vi "Actor Core.vi"(0 "MainUI in":refnum<class "MainUI.lvclass">, 11 "Error in":errorcluster caption="Error in (no error)") -> (4 "MainUI out":refnum<class "MainUI.lvclass">, 15 "Error out":errorcluster)   [LabVIEW 2018, in "HOG MainUI.lvlib" / "MainUI.lvclass"]
doc: "GPower Actor Core VI.\n\nSteen Schmidt\nGPower\n9/9 2018"
uses:
  MainUI.lvclass
  <vilib>/GPower/Actor/Library/Actor Class/Actor.lvclass
  <vilib>/GPower/Actor/Library/Responder Class/Responder.lvclass
  C:/Program Files (x86)/National Instruments/LabVIEW 2018/vi.lib/GPower/Actor/Library/Actor Class/Actor.lvclass
  <vilib>/GPower/UI/Library/GP UI.lvlib
  <vilib>/GPower/UI/Library/Controls/Clear Control/Clear Table.vi
panel:
  in  "MemberList":i32(listbox)
  in  "Search":string
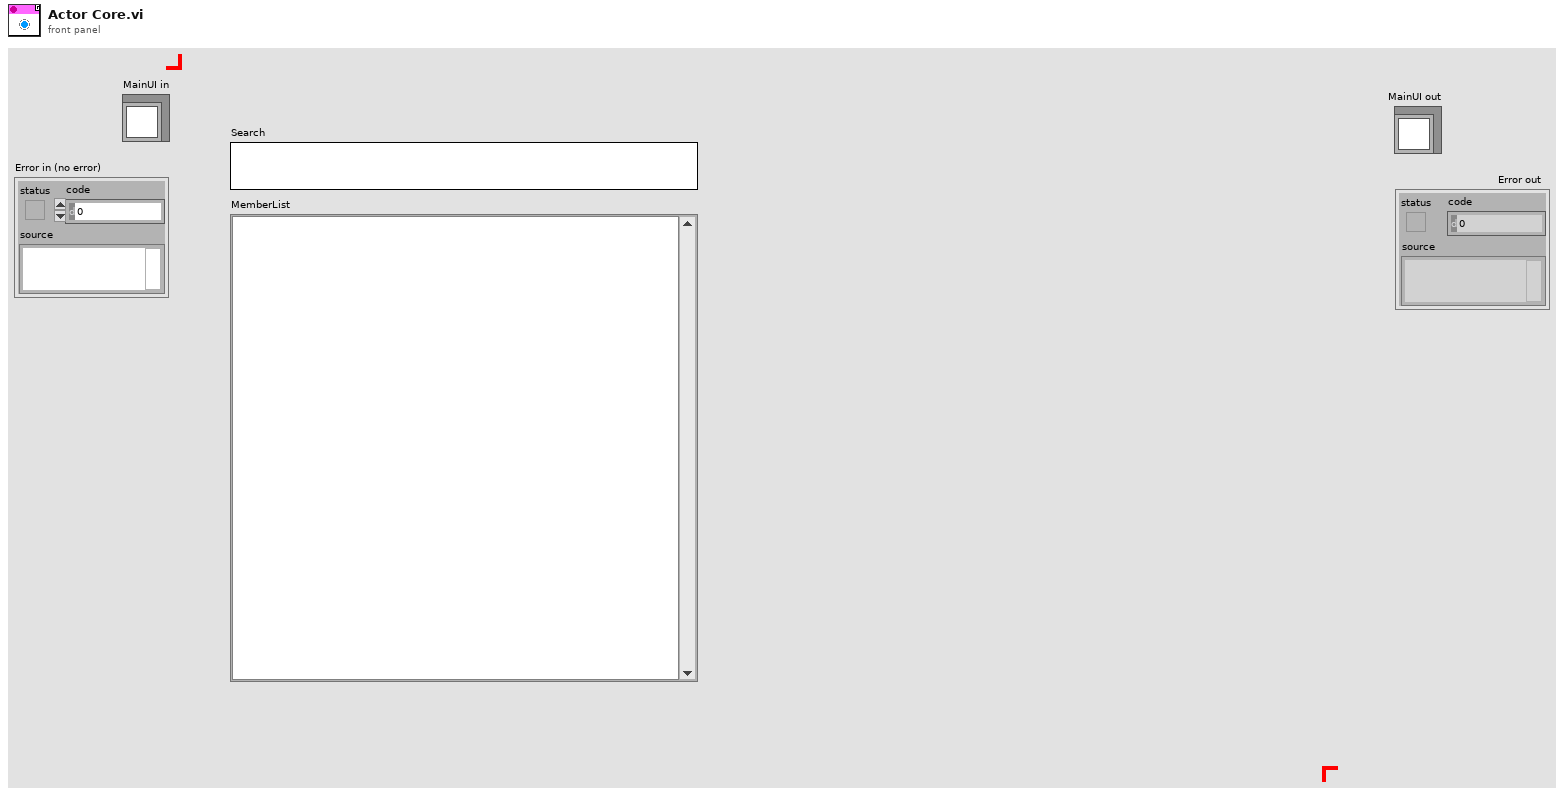
[diagram p1: front panel]
types:
  T1 = typedef "GP Actor.lvlib/Actor Interface.lvclass/Registered Actor Events.ctl" = cluster{"Actor Messages":refnum<event-registration>, "Actor Stopped":refnum<event-registration>, "Actor Stop":refnum<event-registration>}
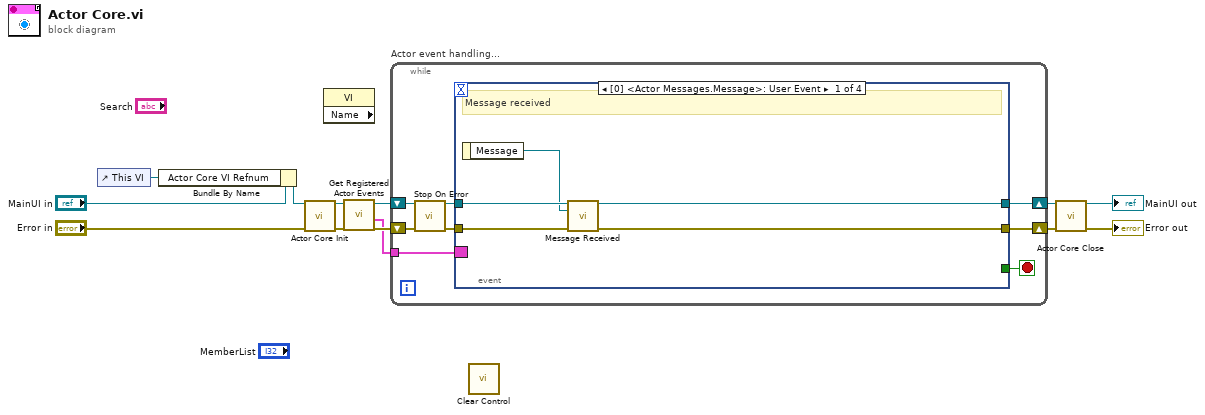
[diagram p0: block diagram]
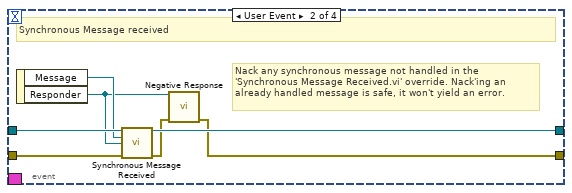
[diagram p2: hidden frame]
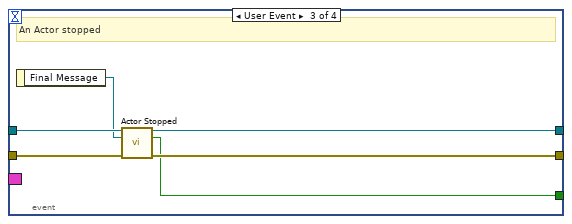
[diagram p3: hidden frame]
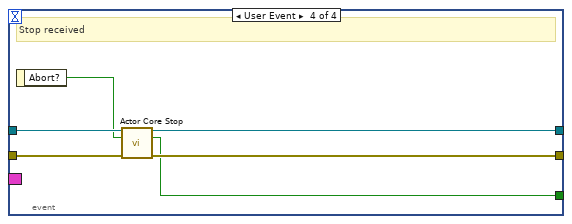
[diagram p4: hidden frame]
diagram:
  n1 = control-ref of="This VI"() -> (w3:refnum<vi>)
  n2 = Bundle By Name(cluster="MainUI in", "Actor Core VI Refnum"=w3) -> (w1:refnum<class "MainUI.lvclass">)
  n3 = call <vilib>:"Actor Core Init.vi"("Actor in"=w1, "Error in"="Error in") -> ("Actor out"=w8:refnum<class "MainUI.lvclass">, "Error out"=w12:errorcluster)  [unwired: 12 in]
  n4 = property class="VI" props=["Name"]() -> ()  [unwired: 2 in, 3 out]
  n5 = call <vilib>:"Get Registered Actor Events.vi"("Actor in"=w8) -> ("Registered Actor Events"=w6:T1, "Actor out"=w7:refnum<class "MainUI.lvclass">)  [unwired: 9 in]
  n6 = while "Actor event handling..." {
    tunnel: w6 -> [w13]
    shift-right: [w19] -> w11
    shift-left: w12 -> [w15]
    shift-right: [w18] -> w10
    shift-left: w7 -> [w17]
    stop <- w20 stop-if-true
    n7 = call <vilib>:"Stop On Error.vi"("Actor in"=w17, "Error in"=w15) -> ("Actor out"=w16:refnum<class "MainUI.lvclass">, "Error out"=w14:errorcluster)  [unwired: 12 in]
    n8 = event shown="[0] <Actor Messages.Message>: User Event" {
      selector: w13 -> [_ _ _ _]
      dyn-events: _ -> [_ _ _ _]
      timeout: _ -> [_ _ _ _]
      tunnel: w16 -> [w25 w30 w37 w44]
      tunnel: w14 -> [w23 w32 w38 w42]
      tunnel: [w22 w27 w36 w41] -> w19
      tunnel: [w24 w31 w35 w43] -> w18
      tunnel: [_ _ w33 w40] -> w20
      event User Event {
        # "Message received"
        n9 = event-data() -> ("Message"=w21:refnum<class "Message.lvclass">)  [unwired: 1 in]
        n10 = call <vilib>:"Message Received.vi"("Actor in"=w25, "Message"=w21, "Error in"=w23) -> ("Actor out"=w24:refnum<class "MainUI.lvclass">, "Error out"=w22:errorcluster)  [unwired: 11 in]
      }
      event User Event {
        # "Nack any synchronous message not handled in the 'Synchronous Message Received.vi' override. Nack'ing an already handled message is safe, it won't yield an error."
        # "Synchronous Message received"
        n11 = event-data() -> ("Message"=w29:refnum<class "Message.lvclass">, "Responder"=w26:refnum<class "Responder.lvclass">)  [unwired: 1 in]
        n12 = call <vilib>:"Synchronous Message Received.vi"("Actor in"=w30, "Message"=w29, "Responder"=w26, "Error in"=w32) -> ("Actor out"=w31:refnum<class "MainUI.lvclass">, "Error out"=w28:errorcluster)  [unwired: 10 in]
        n13 = call <vilib>:"Negative Response.vi"("Responder"=w26, "Error in"=w28) -> ("Error out"=w27:errorcluster)  [unwired: 13 in]
      }
      event User Event {
        # "An Actor stopped"
        n14 = event-data() -> ("Final Message"=w34:refnum<class "Final Message.lvclass">)  [unwired: 1 in]
        n15 = call <vilib>:"Actor Stopped.vi"("Actor in"=w37, "Stopped Actor Final Message"=w34, "Error in"=w38) -> ("Actor out"=w35:refnum<class "MainUI.lvclass">, "Stop Myself Now?"=w33:bool, "Error out"=w36:errorcluster)  [unwired: 10 in]
      }
      event User Event {
        # "Stop received"
        n16 = event-data() -> ("Abort?"=w39:bool)  [unwired: 1 in]
        n17 = call <vilib>:"Actor Core Stop.vi"("Actor in"=w44, "Abort?"=w39, "Error in"=w42) -> ("Actor out"=w43:refnum<class "MainUI.lvclass">, "Stop Myself Now?"=w40:bool, "Error out"=w41:errorcluster)  [unwired: 10 in]
      }
    }
  }
  n18 = call-poly <vilib>:"Clear Control.vi"() -> ()  [unwired: 15 in, 1 out]
  n19 = call <vilib>:"Actor Core Close.vi"("Actor in"=w10, "Error in"=w11) -> ("Actor out"=→"MainUI out":refnum<class "MainUI.lvclass">, "Error out"=→"Error out":errorcluster)  [unwired: 12 in]
